vi "waveform to array.vi"(10 "complex baseband data":waveform(cdb)[](array[waveform])) -> (2 "Y":cdb[](array[numeric]))   [LabVIEW 2020]
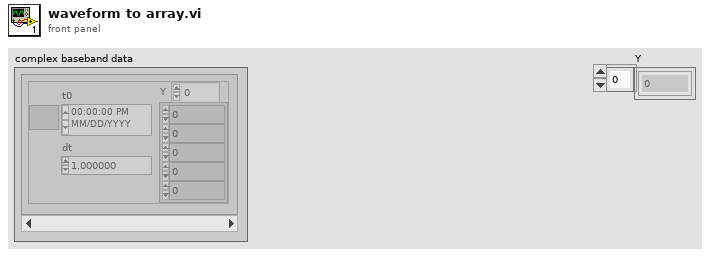
[diagram p1: front panel]
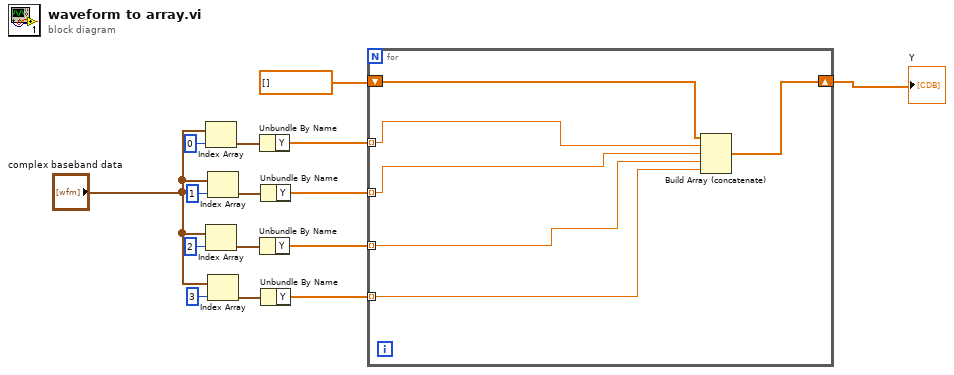
[diagram p0: block diagram]
diagram:
  n1 = Index Array(array="complex baseband data", index=0) -> (element=w10:waveform(cdb))
  n2 = Index Array(array="complex baseband data", index=2) -> (element=w8:waveform(cdb))
  n3 = Index Array(array="complex baseband data", index=1) -> (element=w9:waveform(cdb))
  n4 = Index Array(array="complex baseband data", index=3) -> (element=w7:waveform(cdb))
  n5 = Unbundle By Name(w10) -> ("Y"=w6:cdb[])
  n6 = Unbundle By Name(w8) -> ("Y"=w4:cdb[])
  n7 = Unbundle By Name(w9) -> ("Y"=w5:cdb[])
  n8 = Unbundle By Name(w7) -> ("Y"=w3:cdb[])
  n9 = for {
    tunnel: w6 -> [w20] mode=indexing
    tunnel: w5 -> [w19] mode=indexing
    tunnel: w4 -> [w18] mode=indexing
    tunnel: w3 -> [w17] mode=indexing
    shift-right: [w16] -> w2
    shift-left: cdb[] [] ("Y") -> [w21]
    n10 = Build Array (concatenate)(w21, w20, w19, w18, w17) -> (w16:cdb[])
  }
  "Y" <- w2
